vi "esp_gpib_read_ASCII.vi"(0 "Port In":i32, 1 "Status In":i32, 2 "error in":errorcluster, 3 "Delay In":u16, 4 "Query":bool=TRUE) -> (5 "StringOut":string="0, 3770719, NO ERROR DETECTED\r\n", 6 "Port Out":i32, 7 "Status Out":i32, 8 "error out":errorcluster, 9 "Delay Out":u16)   [LabVIEW 2015]
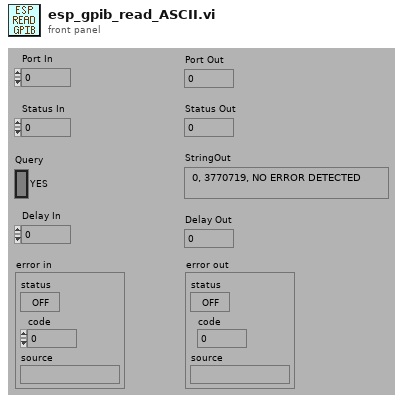
[diagram p1: front panel]
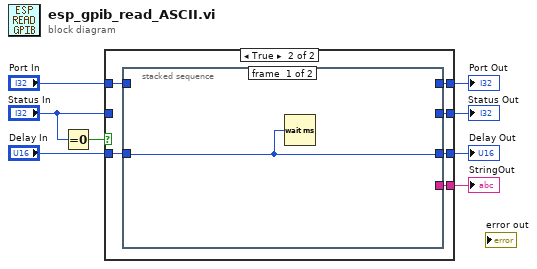
[diagram p0: block diagram]
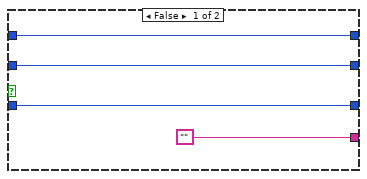
[diagram p2: hidden frame]
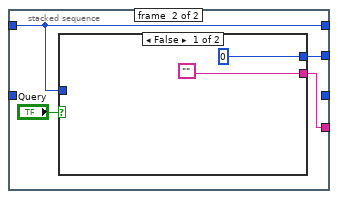
[diagram p3: hidden frame]
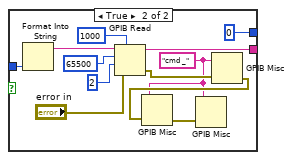
[diagram p4: hidden frame]
diagram:
  n1 = Equal To 0?(x="Status In") -> (x = 0?=w8:bool)
  n2 = case shown="True" w8 {
    tunnel: [w12 w17] -> w7
    tunnel: "Delay In" -> [w12 w18]
    tunnel: "Status In" -> [w11 _]
    tunnel: [w11 w13] -> w4
    tunnel: "Port In" -> [w9 w16]
    tunnel: ["" w15] -> w2
    tunnel: [w9 w14] -> w1
    frame False {
    }
    frame True {
      n3 = stacked-sequence {
        tunnel: w18 -> [w19 _]
        tunnel: [w19 _] -> w17
        tunnel: w16 -> [_ w21]
        tunnel: [_ w20] -> w13
        tunnel: [_ w22] -> w15
        tunnel: [_ w21] -> w14
        frame #0 {
          n4 = Wait (ms)(milliseconds to wait=w19) -> ()  [unwired: 1 out]
        }
        frame #1 {
          n5 = case shown="False" "Query" {
            tunnel: w21 -> [_ w37]
            tunnel: ["" w34] -> w22
            tunnel: [0 0] -> w20
            frame False {
            }
            frame True {
              w26 = "cmd _" ("command string")
              n6 = Format Into String(w37) -> (resulting string=w36:string)  [unwired: 3 in, 1 out]
              n7 = GPIB Read(0:w36, 1:65500 ("byte count"), 2:i16 2 ("mode (0)"), 3:"error in", 4:1000 ("timeout ms (488.2 global)")) -> (5:w34:string, 7:w29:errorcluster)  [unwired: 1 out]
              n8 = GPIB Misc(0:w26, 1:w29) -> (4:w27:errorcluster)  [unwired: 2 out]
              n9 = GPIB Misc(0:w26, 1:w27) -> (4:w28:errorcluster)  [unwired: 2 out]
              n10 = GPIB Misc(0:w26, 1:w28) -> ()  [unwired: 3 out]
            }
          }
        }
      }
    }
  }
  "Delay Out" <- w7
  "Status Out" <- w4
  "StringOut" <- w2
  "Port Out" <- w1
